vi "OP_Print_TPS20161119.vi"() -> ()   [LabVIEW 2013]
uses:
  <userlib>/caLab/Private/Get_PV-1D.vi
  <userlib>/caLab/Private/Get_PV.vi
panel:
  in  "Radio Buttons 2":enum32{"absolute", "different with"}(radio)=enum."different with"
  out "BPMY Graph":cluster{i32[], "1rst Value (number)":dbl[]}(graph)
  out "BPMX Graph":cluster{i32[], "1rst Value (number)":dbl[]}(graph)
  out "date (last Gun ON)":string="2016/08/29"
  out "time string (last Gun ON)":string="23:28:50"
  out "time string (last kicker ON)":string="23:28:50"
  out "date (last kicker ON)":string="2016/08/29"
  out "date":string="2016/08/29"
  out "time string":string="23:28:50"
  out "FOFB V":string="MBM"
  out "FOFB H":string="MBM"
  out "Value Array (number) 7":dbl[](array[numeric])=[7.29, 8.074, 40.001, 7.0, 11.0, 8.18, 40.0, 64.99985000000001, 0.0001, 65.00399999999999, 0.00055, 44.9999, 0.00025, -1.0899999999999999, 130.00060000000002]
  out "45XBPMY 1":dbl format="%#.2f"
  out "41XBPMY 1":dbl format="%#.2f"
  out "25XBPMY 1":dbl format="%#.2f"
  out "23XBPMY 1":dbl format="%#.2f"
  out "21XBPMY 1":dbl format="%#.2f"
  out "09XBPMY 1":dbl format="%#.2f"
  out "05XBPMY 1":dbl format="%#.2f"
  out "45XBPMX 1":dbl format="%#.2f"
  out "41XBPMX 1":dbl format="%#.2f"
  out "Value Array (number) 6":dbl[](array[numeric])=[7.29, 8.074, 40.001, 7.0, 11.0, 8.18, 40.0, 64.99985000000001, 0.0001, 65.00399999999999, 0.00055, 44.9999, 0.00025, -1.0899999999999999, 130.00060000000002]
  out "1rst Value (string) 2":string[](array[string])=["MBM", "33", "23.5", "350", "35.8", "22485", "22485", "62", "30", "0", "0", "160", "100"]
  out "Value Array (number) 5":dbl[](array[numeric])=[499654641.19275105, 1.0, 0.0, 1335.005102558433, 1400.0, -56.1, 1.0, 0.0, 1362.1066276040413, 1400.0, 160.0]
  out "1rst Value (string)":string[](array[string])=["Linac2016_1005_0935.data", "LTB_JT_2016_1005_1200.data", "Booster_JT_2016_1005_1200.data", "BTS_2016_1116_1020.data", "SR_DMB_2016_1102_1124LOCO.data"]
  out "Value Array (number) 4":dbl[](array[numeric])=[499654659.7918481, 1.0, 0.0, 1334.3992420266973, 1400.0, -56.70000000000001, 1.0, 0.0, 1364.2963125179533, 1400.0, 160.0]
  out "Value Array (number) 3":dbl[](array[numeric])=[0.0, 33.0, 23.5, 350.0, 35.800000000000026, 22485.0, 22485.0, 62.0, 30.0, 0.0, 0.0, 160.0, 100.0]
  out "Value Array (number) 2":dbl[](array[numeric])=[105.2, 16.40000000000001, 18.266, 18.26600000000001, 318.8444, 444.5, 419.3416, 417.0, 8.4, 8.325, 8.315, 8.27]
  out "Value Array (number)":dbl[](array[numeric])=[1.0, 302.073574, 665.9266107283645, 46.49677486881546, 27.851792365219392, 0.14677103718199608, 0.22504892367906065, 103.0465316772461, 145.84446716308594, 100.0, 630.0, 10.0]
  out "25XBPMX 1":dbl format="%#.2f"
  out "23XBPMX 1":dbl format="%#.2f"
  out "21XBPMX 1":dbl format="%#.2f"
  out "09XBPMX 1":dbl format="%#.2f"
  out "05XBPMX 1":dbl format="%#.2f"
  out "Taper":dbl=-1.0899999999999999 format="%#.4f"
  out "phase shifter":dbl=130.00060000000002 format="%#.3f"
  out "10ps delay":dbl=100.0 format="%#.1f"
  out "2ns step":dbl format="%#.1f"
  out "Width count":dbl=30.0 format="%#.1f"
  out "Gun volt.(S)":dbl=23.5 format="%#.1f"
  out "EPU46-45pM":bool
  out "EPU48B-41pM":bool
  out "EPU48A-41pM":bool
  out "IU22-05 FE Enable":bool=TRUE
  out "IU22A-09 FE Enable":bool=TRUE
  out "IUT22-21 FE Enable":bool=TRUE
  out "IU22-23 FE Enable":bool
  out "IU22A-25 FE Enable":bool=TRUE
  out "EPU48A-41 FE Enable":bool
  out "EPU46-45 FE Enable":bool=TRUE
  out "EPU46-45M Hutch Enable":bool=TRUE
  out "EPU48A-41M Hutch Enable":bool
  out "IU22A-25M Hutch Enable":bool=TRUE
  out "IU22-23M Hutch Enable":bool
  out "IUT22-21M Hutch Enable":bool=TRUE
  out "IU22A-09M Hutch Enable":bool=TRUE
  out "IU22-05 Hutch Enable":bool=TRUE
  out "Orbit ILK(P)":bool
  out "Orbit ILK(A)":bool
  out "Bucket Step":dbl=10.0 format="%#.2f"
  out "Bucket Last":dbl=630.0 format="%#.2f"
  out "Bucket Start":dbl=100.0 format="%#.2f"
  out "Orbit INT. Ang Active":bool
  out "Orbit INT.Ang. On":bool
  out "Orbit INT. Pos Active":bool
  out "Orbit INT.Pos. On":bool
  out "BR ext. kicker1":dbl=18.266 format="%#.2f"
  out "BR ext. kicker2":dbl=18.26600000000001 format="%#.2f"
  out "BR ext. sep.1":dbl=318.8444 format="%#.2f"
  out "BR ext. sep.2":dbl=444.5 format="%#.2f"
  out "BR inj. sep.":dbl=105.2 format="%#.3f"
  out "BR inj. kicker":dbl=16.40000000000001 format="%#.3f"
  out "SR kicker4":dbl=8.27 format="%#.2f"
  out "SR kicker3":dbl=8.315 format="%#.2f"
  out "SR kicker2":dbl=8.325 format="%#.2f"
  out "SR kicker1":dbl=8.4 format="%#.2f"
  out "SR inj. sep.2":dbl=417.0 format="%#.2f"
  out "SR inj. sep.1":dbl=419.3416 format="%#.2f"
  out "BBF H":bool
  out "BBF V":bool
  out "RF3 gap volt.(S)":dbl=1400.0 format="%#.0f"
  out "RF3 phase.(S)":dbl=160.0 format="%#.0f"
  out "RF3 OP mode":bool=TRUE
  out "RF3 remote":bool=TRUE
  out "RF2 gap volt.(S)":dbl=1400.0 format="%#.0f"
  out "RF Freq.(s)":dbl=499654659.7918481 format="%#.1f"
  out "RF2 phase.(S)":dbl=-56.70000000000001 format="%#.0f"
  out "RF2 OP mode":bool=TRUE
  out "RF2 remote":bool=TRUE
  out "BTS":string="SR_DMB_2016_1102_1124LOCO.data"
  out "LTB":string="LTB_JT_2016_1005_1200.data"
  out "Linac":string="Linac2016_1005_0935.data"
  out "BR":string="BTS_2016_1116_1020.data"
  out "SR":string="Booster_JT_2016_1005_1200.data"
  out "Mod.3 HV(S)":dbl=35.800000000000026 format="%#.1f"
  out "SBM volt.(S)":dbl=350.0 format="%#.1f"
  out "MBM volt.(S)":dbl=23.5 format="%#.1f"
  out "Gun mode":string="MBM"
  out "Grid volt.(S)":dbl=33.0 format="%#.1f"
  out "EPU46-45phase(R)":dbl=0.00025 format="%#.4f"
  out "EPU48B-41phase(R)":dbl=0.00055 format="%#.4f"
  out "EPU48A-41phase(R)":dbl=0.0001 format="%#.4f"
  out "EPU46-45gM":bool
  out "EPU46-45gap(R)":dbl=44.9999 format="%#.4f"
  out "EPU48B-41gM":bool
  out "EPU48B-41gap(R)":dbl=65.00399999999999 format="%#.4f"
  out "EPU48A-41gM":bool
  out "EPU48A-41gap(R)":dbl=64.99985000000001 format="%#.4f"
  out "IU22B-25M":bool
  out "IU22B-25gap(R)":dbl=40.0 format="%#.4f"
  out "IU22A-25M":bool
  out "IU22A-25gap(R)":dbl=8.18 format="%#.4f"
  out "IU22-23M":bool
  out "IUT22-21M":bool
  out "IUT22-21gap(R)":dbl=7.0 format="%#.4f"
  out "IU22B-09M":bool
  out "IU22B-09gap(R)":dbl=40.001 format="%#.4f"
  out "IU22A-09M":bool
  out "IU22A-09gap(R)":dbl=8.074 format="%#.4f"
  out "IU22-05M":bool
  out "IU22-05gap(R)":dbl=7.29 format="%#.4f"
  out "IU22-23gap(R)":dbl=11.0 format="%#.4f"
  out "NuY(form BBF)":dbl=0.25219386232318686 format="%#.2f"
  out "NuX(form BBF)":dbl=0.1781877868128751 format="%#.2f"
  out "Mode":string="Top-Up"
  out "Tune Y(form BPM)":dbl=0.2162426614481409 format="%#.2f"
  out "Tune X(form BPM)":dbl=0.14677103718199608 format="%#.2f"
  out "Beamsize Y(um)":dbl=33.47785442299371 format="%#.2f"
  out "Beamsize X(um)":dbl=55.88912339231618 format="%#.2f"
  out "Beam Lifetime(min)":dbl=665.9266107283645 format="%#.3f"
  out "Beam Current(mA":dbl=302.073574 format="%#.3f"
  in  "Copy Button":bool
  in  "Print Button":bool
  in  "Help Button":bool
  in  "Refresh Button":bool
  in  "Open Button":bool
  out "Gun WCM":dbl[](graph)
  out "BR Fill Pattern":dbl[](graph)
  out "SR Fill Pattern":dbl[](graph)
  # "Valve  Status"
  # "TPS OP Handover Information"
  # "SM Status"
  # "TPS Operational Handover Information v1.0"
  # "Time："
  # "Others"
  # "SR Status"
  # "Feedback"
  # "Pulse Mag. Status"
  # "LINAC Status"
  # "RF Status"
  # "Hz"
  # "Changeliang@BD.NSRRC"
  # "SR Fill Pattern"
  # "Lattice Files in using"
  # "歷史電流圖\ntrip次數?\n輻射劑量?\n平均氣壓\n目前最高累計劑量\n最近一次觸發時BR電流及WCM數值"
  # "ID &Beamline Status"
  # "Gap"
  # "Motor"
  # "Phase"
  # "FE/Hutch"
  # "phase\nshifter"
  # "Taper"
  # "XBPM1X\num"
  # "XBPM1Y\num"
  # "05"
  # "09"
  # "21"
  # "23"
  # "25"
  # "41"
  # "45"
  # "SR Orbit"
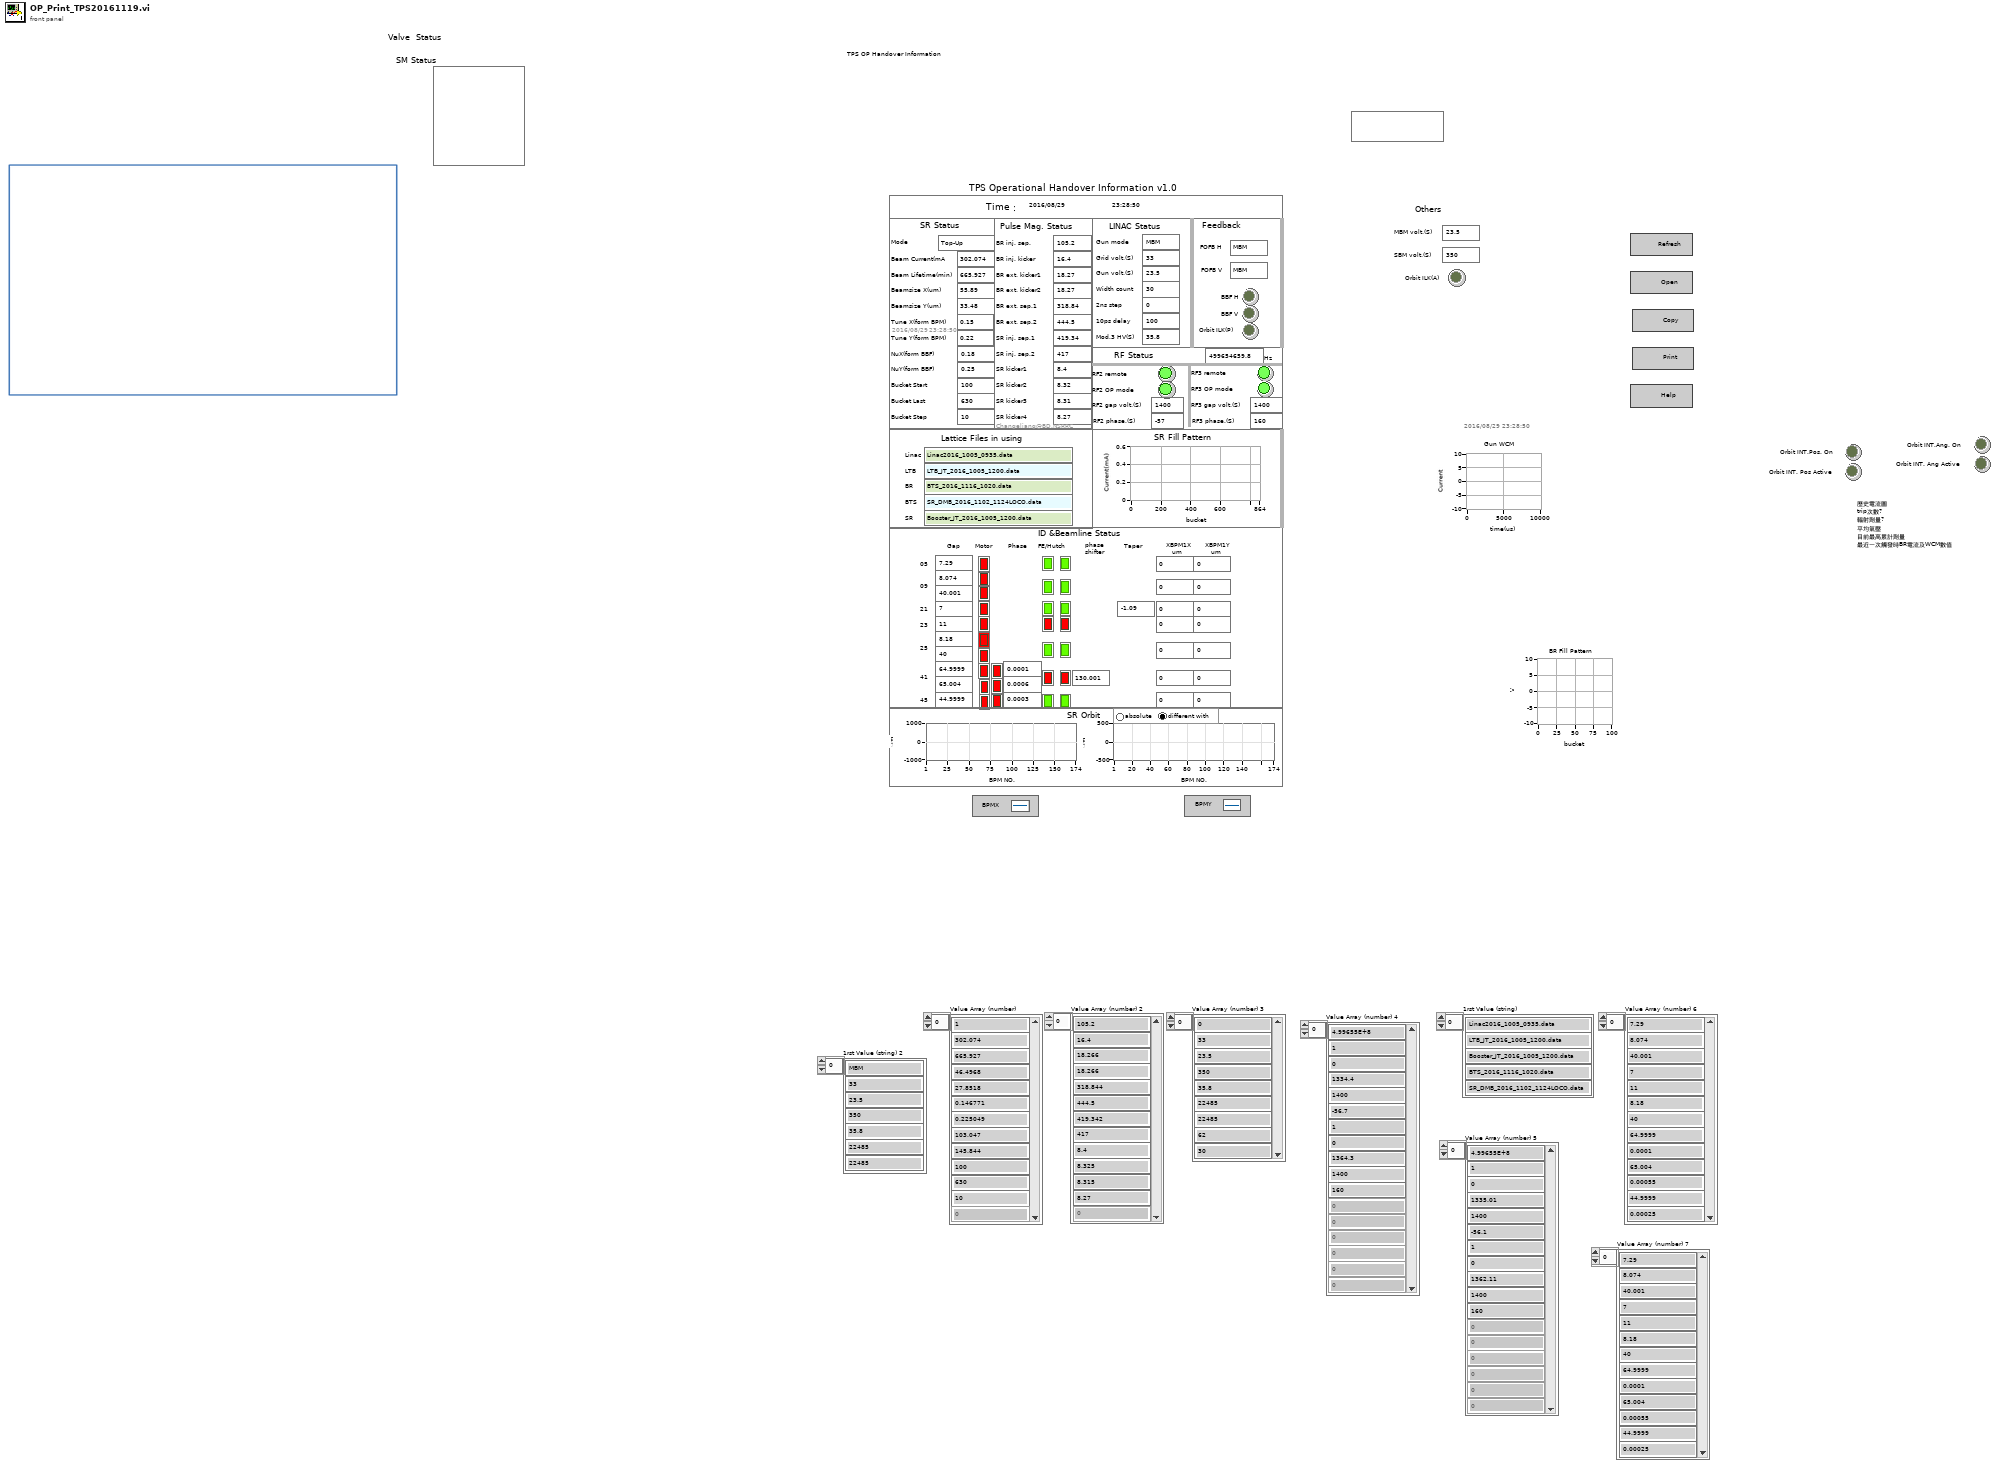
[diagram p1: front panel]
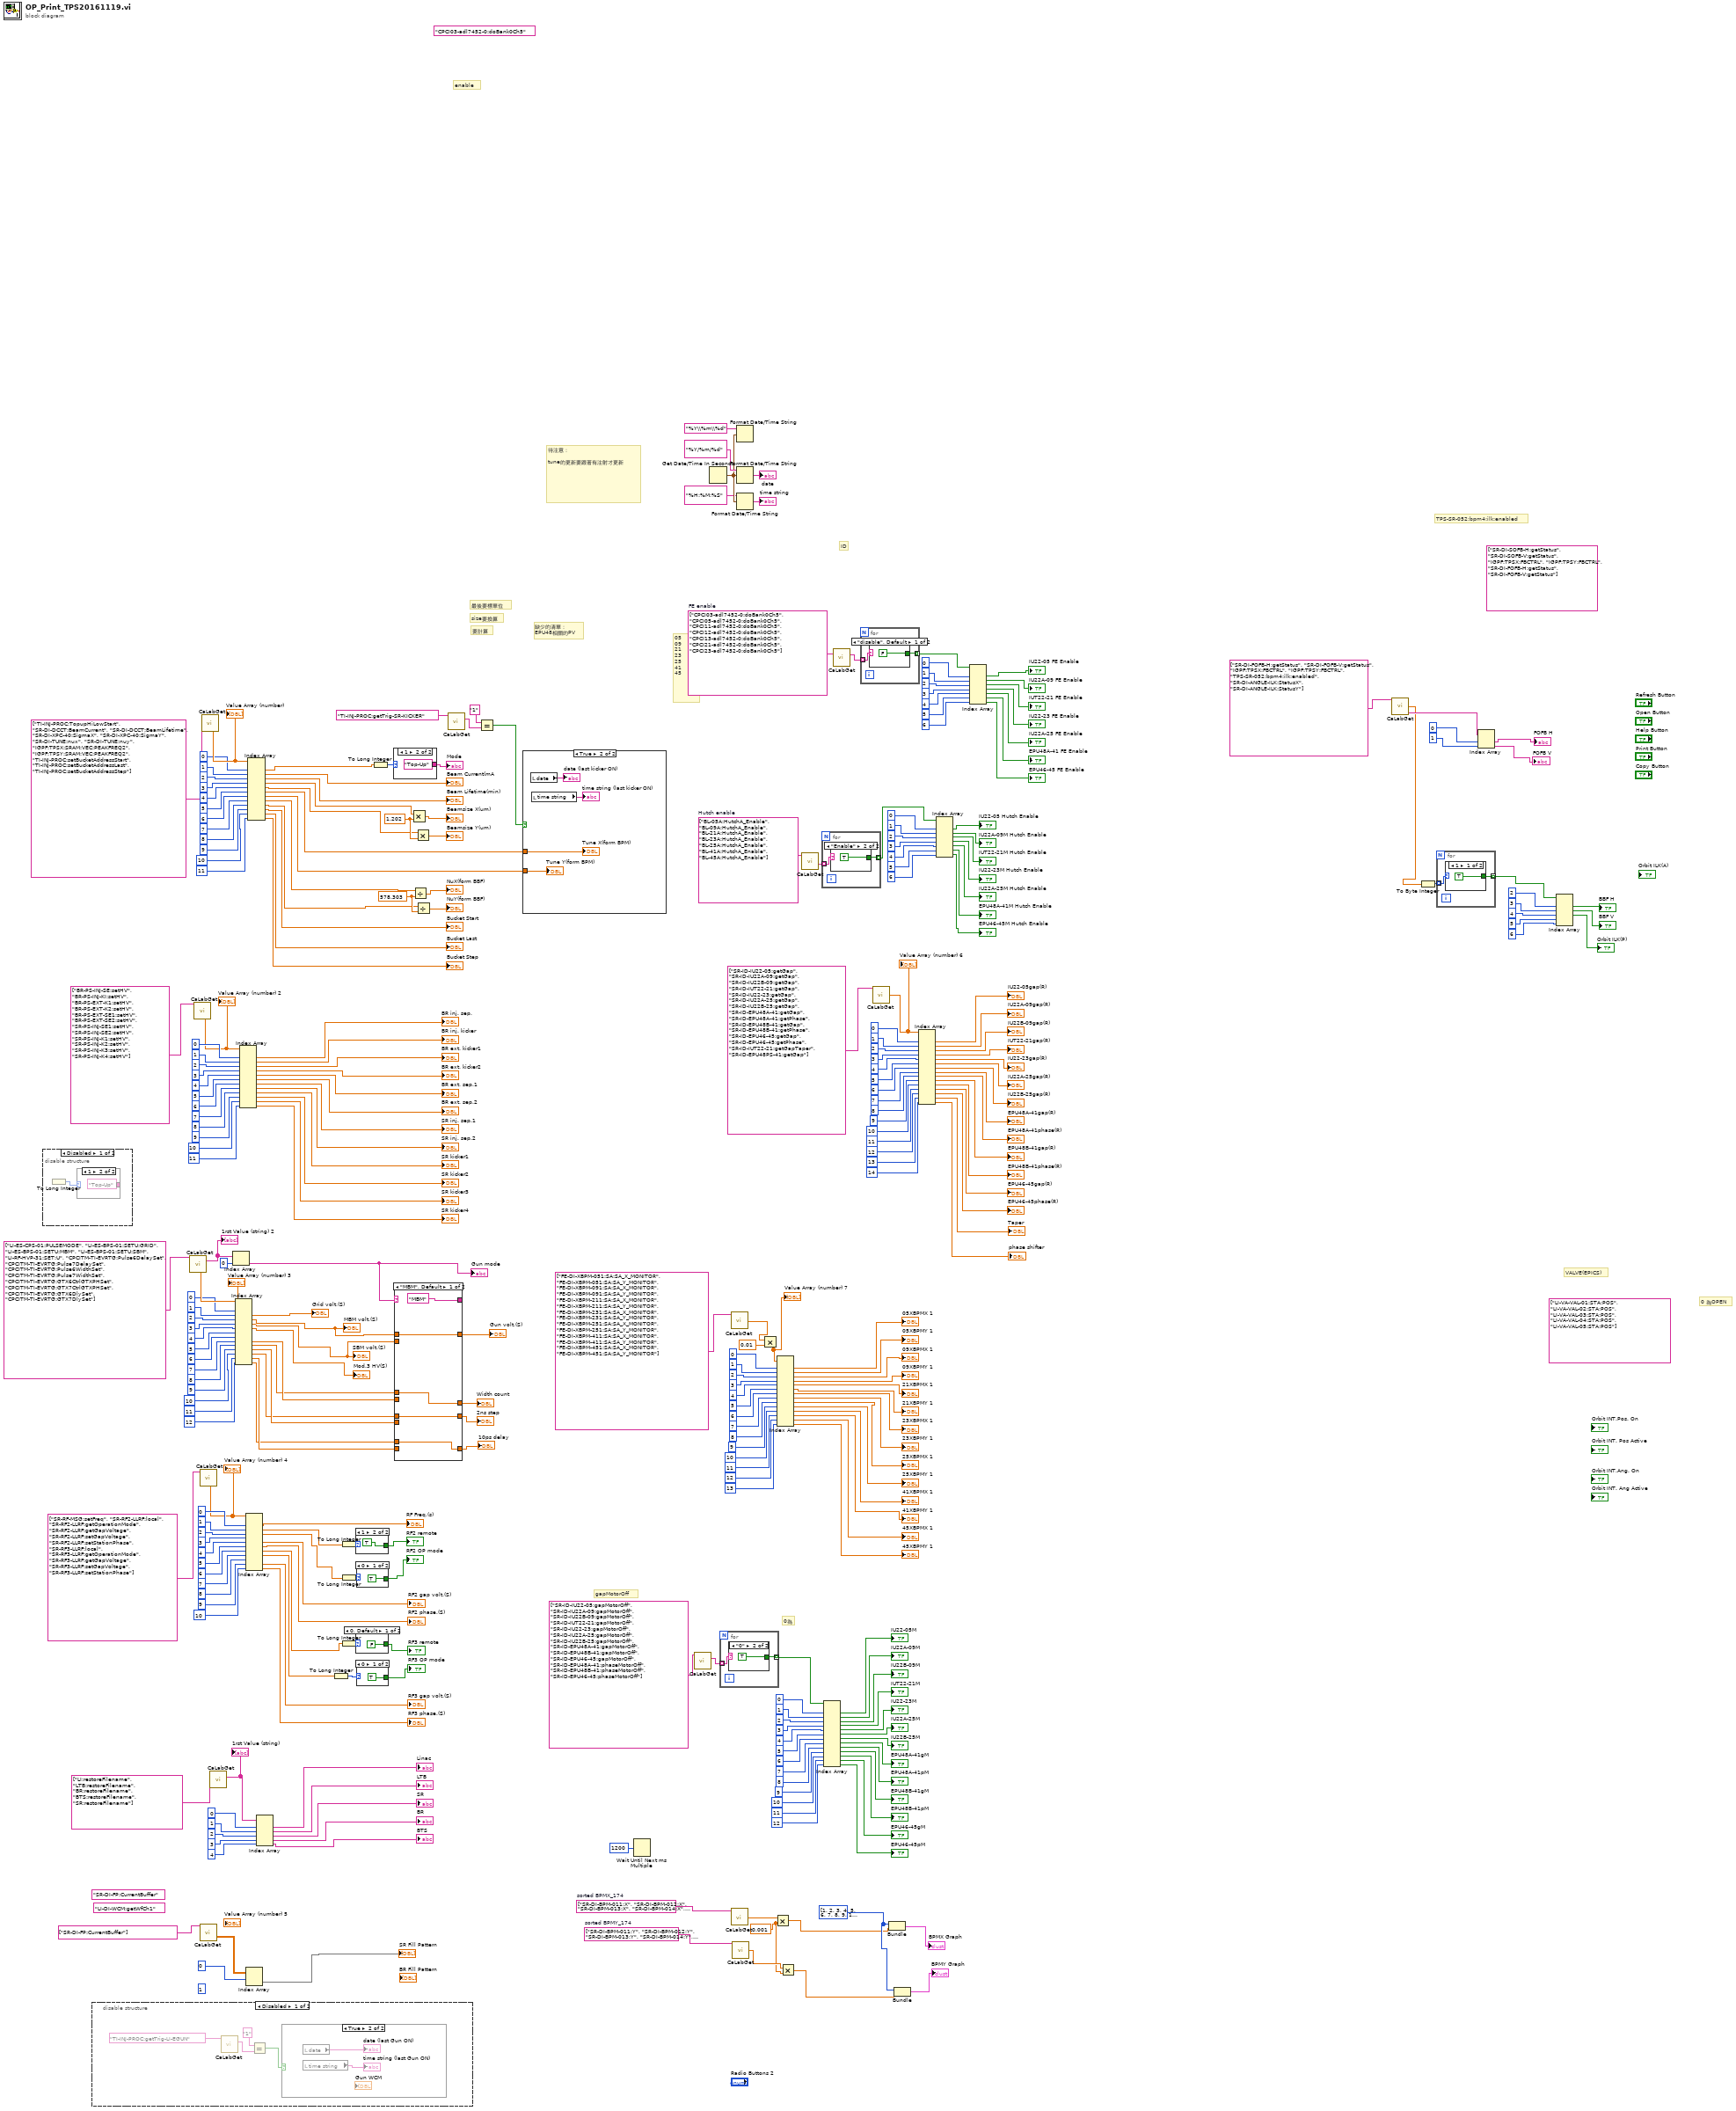
[diagram p0: block diagram]
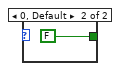
[diagram p4: hidden frame]
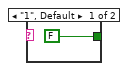
[diagram p5: hidden frame]
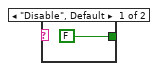
[diagram p6: hidden frame]
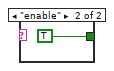
[diagram p7: hidden frame]
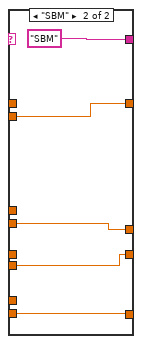
[diagram p8: hidden frame]
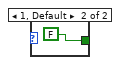
[diagram p10: hidden frame]
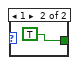
[diagram p11: hidden frame]
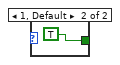
[diagram p12: hidden frame]
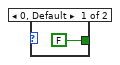
[diagram p13: hidden frame]
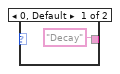
[diagram p14: hidden frame]
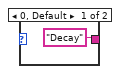
[diagram p16: hidden frame]
diagram:
  (unwired) "LI-DI-WCM:getWfCh1"
  (unwired) "SR-DI-FP:CurrentBuffer"
  w12 = i32[] [1, 2, 3, 4, 5, 6, 7, 8, 9, 10, 11, 12, 13, 14, 15, 16, 17, 18, 19, 20, 21, 22, 23, 24, 25, 26, 27, 28, 29, 30, 31, 32, 33, 34, 35, 36, 37, 38, 39, 40, 41, 42, 43, 44, 45, 46, 47, 48, 49, 50, 51, 52, 53, 54, 55, 56, 57, 58, 59, 60, 61, 62, 63, 64, 65, 66, 67, 68, 69, 70, 71, 72, 73, 74, 75, 76, 77, 78, 79, 80, 81, 82, 83, 84, 85, 86, 87, 88, 89, 90, 91, 92, 93, 94, 95, 96, 97, 98, 99, 100, 101, 102, 103, 104, 105, 106, 107, 108, 109, 110, 111, 112, 113, 114, 115, 116, 117, 118, 119, 120, 121, 122, 123, 124, 125, 126, 127, 128, 129, 130, 131, 132, 133, 134, 135, 136, 137, 138, 139, 140, 141, 142, 143, 144, 145, 146, 147, 148, 149, 150, 151, 152, 153, 154, 155, 156, 157, 158, 159, 160, 161, 162, 163, 164, 165, 166, 167, 168, 169, 170, 171, 172, 173, 174] ("Array 4")
  w9 = 0.001
  w6 = string[] ["SR-DI-BPM-011:Y", "SR-DI-BPM-012:Y", "SR-DI-BPM-013:Y", "SR-DI-BPM-014:Y", "SR-DI-BPM-015:Y", "SR-DI-BPM-016:Y", "SR-DI-BPM-017:Y", "SR-DI-BPM-021:Y", "SR-DI-BPM-022:Y", "SR-DI-BPM-023:Y", "SR-DI-BPM-024:Y", "SR-DI-BPM-025:Y", "SR-DI-BPM-026:Y", "SR-DI-BPM-027:Y", "SR-DI-BPM-031:Y", "SR-DI-BPM-032:Y", "SR-DI-BPM-033:Y", "SR-DI-BPM-034:Y", "SR-DI-BPM-035:Y", "SR-DI-BPM-036:Y", "SR-DI-BPM-037:Y", "SR-DI-BPM-041:Y", "SR-DI-BPM-042:Y", "SR-DI-BPM-043:Y", "SR-DI-BPM-044:Y", "SR-DI-BPM-045:Y", "SR-DI-BPM-046:Y", "SR-DI-BPM-047:Y", "SR-DI-BPM-048:Y", "SR-DI-BPM-050:Y", "SR-DI-BPM-051:Y", "SR-DI-BPM-052:Y", "SR-DI-BPM-053:Y", "SR-DI-BPM-054:Y", "SR-DI-BPM-055:Y", "SR-DI-BPM-056:Y", "SR-DI-BPM-057:Y", "SR-DI-BPM-061:Y", "SR-DI-BPM-062:Y", "SR-DI-BPM-063:Y", "SR-DI-BPM-064:Y", "SR-DI-BPM-065:Y", "SR-DI-BPM-066:Y", "SR-DI-BPM-067:Y", "SR-DI-BPM-071:Y", "SR-DI-BPM-072:Y", "SR-DI-BPM-073:Y", "SR-DI-BPM-074:Y", "SR-DI-BPM-075:Y", "SR-DI-BPM-076:Y", "SR-DI-BPM-077:Y", "SR-DI-BPM-081:Y", "SR-DI-BPM-082:Y", "SR-DI-BPM-083:Y", "SR-DI-BPM-084:Y", "SR-DI-BPM-085:Y", "SR-DI-BPM-086:Y", "SR-DI-BPM-087:Y", "SR-DI-BPM-091:Y", "SR-DI-BPM-092:Y", "SR-DI-BPM-093:Y", "SR-DI-BPM-094:Y", "SR-DI-BPM-095:Y", "SR-DI-BPM-096:Y", "SR-DI-BPM-097:Y", "SR-DI-BPM-101:Y", "SR-DI-BPM-102:Y", "SR-DI-BPM-103:Y", "SR-DI-BPM-104:Y", "SR-DI-BPM-105:Y", "SR-DI-BPM-106:Y", "SR-DI-BPM-107:Y", "SR-DI-BPM-111:Y", "SR-DI-BPM-112:Y", "SR-DI-BPM-113:Y", "SR-DI-BPM-114:Y", "SR-DI-BPM-115:Y", "SR-DI-BPM-116:Y", "SR-DI-BPM-117:Y", "SR-DI-BPM-121:Y", "SR-DI-BPM-122:Y", "SR-DI-BPM-123:Y", "SR-DI-BPM-124:Y", "SR-DI-BPM-125:Y", "SR-DI-BPM-126:Y", "SR-DI-BPM-127:Y", "SR-DI-BPM-128:Y", "SR-DI-BPM-130:Y", "SR-DI-BPM-131:Y", "SR-DI-BPM-132:Y", "SR-DI-BPM-133:Y", "SR-DI-BPM-134:Y", "SR-DI-BPM-135:Y", "SR-DI-BPM-136:Y", "SR-DI-BPM-137:Y", "SR-DI-BPM-141:Y", "SR-DI-BPM-142:Y", "SR-DI-BPM-143:Y", "SR-DI-BPM-144:Y", "SR-DI-BPM-145:Y", "SR-DI-BPM-146:Y", "SR-DI-BPM-147:Y", "SR-DI-BPM-151:Y", "SR-DI-BPM-152:Y", "SR-DI-BPM-153:Y", "SR-DI-BPM-154:Y", "SR-DI-BPM-155:Y", "SR-DI-BPM-156:Y", "SR-DI-BPM-157:Y", "SR-DI-BPM-161:Y", "SR-DI-BPM-162:Y", "SR-DI-BPM-163:Y", "SR-DI-BPM-164:Y", "SR-DI-BPM-165:Y", "SR-DI-BPM-166:Y", "SR-DI-BPM-167:Y", "SR-DI-BPM-171:Y", "SR-DI-BPM-172:Y", "SR-DI-BPM-173:Y", "SR-DI-BPM-174:Y", "SR-DI-BPM-175:Y", "SR-DI-BPM-176:Y", "SR-DI-BPM-177:Y", "SR-DI-BPM-181:Y", "SR-DI-BPM-182:Y", "SR-DI-BPM-183:Y", "SR-DI-BPM-184:Y", "SR-DI-BPM-185:Y", "SR-DI-BPM-186:Y", "SR-DI-BPM-187:Y", "SR-DI-BPM-191:Y", "SR-DI-BPM-192:Y", "SR-DI-BPM-193:Y", "SR-DI-BPM-194:Y", "SR-DI-BPM-195:Y", "SR-DI-BPM-196:Y", "SR-DI-BPM-197:Y", "SR-DI-BPM-201:Y", "SR-DI-BPM-202:Y", "SR-DI-BPM-203:Y", "SR-DI-BPM-204:Y", "SR-DI-BPM-205:Y", "SR-DI-BPM-206:Y", "SR-DI-BPM-207:Y", "SR-DI-BPM-208:Y", "SR-DI-BPM-210:Y", "SR-DI-BPM-211:Y", "SR-DI-BPM-212:Y", "SR-DI-BPM-213:Y", "SR-DI-BPM-214:Y", "SR-DI-BPM-215:Y", "SR-DI-BPM-216:Y", "SR-DI-BPM-217:Y", "SR-DI-BPM-221:Y", "SR-DI-BPM-222:Y", "SR-DI-BPM-223:Y", "SR-DI-BPM-224:Y", "SR-DI-BPM-225:Y", "SR-DI-BPM-226:Y", "SR-DI-BPM-227:Y", "SR-DI-BPM-231:Y", "SR-DI-BPM-232:Y", "SR-DI-BPM-233:Y", "SR-DI-BPM-234:Y", "SR-DI-BPM-235:Y", "SR-DI-BPM-236:Y", "SR-DI-BPM-237:Y", "SR-DI-BPM-241:Y", "SR-DI-BPM-242:Y", "SR-DI-BPM-243:Y", "SR-DI-BPM-244:Y", "SR-DI-BPM-245:Y", "SR-DI-BPM-246:Y", "SR-DI-BPM-247:Y"]  # sorted BPMY_174
  w5 = string[] ["SR-DI-BPM-011:X", "SR-DI-BPM-012:X", "SR-DI-BPM-013:X", "SR-DI-BPM-014:X", "SR-DI-BPM-015:X", "SR-DI-BPM-016:X", "SR-DI-BPM-017:X", "SR-DI-BPM-021:X", "SR-DI-BPM-022:X", "SR-DI-BPM-023:X", "SR-DI-BPM-024:X", "SR-DI-BPM-025:X", "SR-DI-BPM-026:X", "SR-DI-BPM-027:X", "SR-DI-BPM-031:X", "SR-DI-BPM-032:X", "SR-DI-BPM-033:X", "SR-DI-BPM-034:X", "SR-DI-BPM-035:X", "SR-DI-BPM-036:X", "SR-DI-BPM-037:X", "SR-DI-BPM-041:X", "SR-DI-BPM-042:X", "SR-DI-BPM-043:X", "SR-DI-BPM-044:X", "SR-DI-BPM-045:X", "SR-DI-BPM-046:X", "SR-DI-BPM-047:X", "SR-DI-BPM-048:X", "SR-DI-BPM-050:X", "SR-DI-BPM-051:X", "SR-DI-BPM-052:X", "SR-DI-BPM-053:X", "SR-DI-BPM-054:X", "SR-DI-BPM-055:X", "SR-DI-BPM-056:X", "SR-DI-BPM-057:X", "SR-DI-BPM-061:X", "SR-DI-BPM-062:X", "SR-DI-BPM-063:X", "SR-DI-BPM-064:X", "SR-DI-BPM-065:X", "SR-DI-BPM-066:X", "SR-DI-BPM-067:X", "SR-DI-BPM-071:X", "SR-DI-BPM-072:X", "SR-DI-BPM-073:X", "SR-DI-BPM-074:X", "SR-DI-BPM-075:X", "SR-DI-BPM-076:X", "SR-DI-BPM-077:X", "SR-DI-BPM-081:X", "SR-DI-BPM-082:X", "SR-DI-BPM-083:X", "SR-DI-BPM-084:X", "SR-DI-BPM-085:X", "SR-DI-BPM-086:X", "SR-DI-BPM-087:X", "SR-DI-BPM-091:X", "SR-DI-BPM-092:X", "SR-DI-BPM-093:X", "SR-DI-BPM-094:X", "SR-DI-BPM-095:X", "SR-DI-BPM-096:X", "SR-DI-BPM-097:X", "SR-DI-BPM-101:X", "SR-DI-BPM-102:X", "SR-DI-BPM-103:X", "SR-DI-BPM-104:X", "SR-DI-BPM-105:X", "SR-DI-BPM-106:X", "SR-DI-BPM-107:X", "SR-DI-BPM-111:X", "SR-DI-BPM-112:X", "SR-DI-BPM-113:X", "SR-DI-BPM-114:X", "SR-DI-BPM-115:X", "SR-DI-BPM-116:X", "SR-DI-BPM-117:X", "SR-DI-BPM-121:X", "SR-DI-BPM-122:X", "SR-DI-BPM-123:X", "SR-DI-BPM-124:X", "SR-DI-BPM-125:X", "SR-DI-BPM-126:X", "SR-DI-BPM-127:X", "SR-DI-BPM-128:X", "SR-DI-BPM-130:X", "SR-DI-BPM-131:X", "SR-DI-BPM-132:X", "SR-DI-BPM-133:X", "SR-DI-BPM-134:X", "SR-DI-BPM-135:X", "SR-DI-BPM-136:X", "SR-DI-BPM-137:X", "SR-DI-BPM-141:X", "SR-DI-BPM-142:X", "SR-DI-BPM-143:X", "SR-DI-BPM-144:X", "SR-DI-BPM-145:X", "SR-DI-BPM-146:X", "SR-DI-BPM-147:X", "SR-DI-BPM-151:X", "SR-DI-BPM-152:X", "SR-DI-BPM-153:X", "SR-DI-BPM-154:X", "SR-DI-BPM-155:X", "SR-DI-BPM-156:X", "SR-DI-BPM-157:X", "SR-DI-BPM-161:X", "SR-DI-BPM-162:X", "SR-DI-BPM-163:X", "SR-DI-BPM-164:X", "SR-DI-BPM-165:X", "SR-DI-BPM-166:X", "SR-DI-BPM-167:X", "SR-DI-BPM-171:X", "SR-DI-BPM-172:X", "SR-DI-BPM-173:X", "SR-DI-BPM-174:X", "SR-DI-BPM-175:X", "SR-DI-BPM-176:X", "SR-DI-BPM-177:X", "SR-DI-BPM-181:X", "SR-DI-BPM-182:X", "SR-DI-BPM-183:X", "SR-DI-BPM-184:X", "SR-DI-BPM-185:X", "SR-DI-BPM-186:X", "SR-DI-BPM-187:X", "SR-DI-BPM-191:X", "SR-DI-BPM-192:X", "SR-DI-BPM-193:X", "SR-DI-BPM-194:X", "SR-DI-BPM-195:X", "SR-DI-BPM-196:X", "SR-DI-BPM-197:X", "SR-DI-BPM-201:X", "SR-DI-BPM-202:X", "SR-DI-BPM-203:X", "SR-DI-BPM-204:X", "SR-DI-BPM-205:X", "SR-DI-BPM-206:X", "SR-DI-BPM-207:X", "SR-DI-BPM-208:X", "SR-DI-BPM-210:X", "SR-DI-BPM-211:X", "SR-DI-BPM-212:X", "SR-DI-BPM-213:X", "SR-DI-BPM-214:X", "SR-DI-BPM-215:X", "SR-DI-BPM-216:X", "SR-DI-BPM-217:X", "SR-DI-BPM-221:X", "SR-DI-BPM-222:X", "SR-DI-BPM-223:X", "SR-DI-BPM-224:X", "SR-DI-BPM-225:X", "SR-DI-BPM-226:X", "SR-DI-BPM-227:X", "SR-DI-BPM-231:X", "SR-DI-BPM-232:X", "SR-DI-BPM-233:X", "SR-DI-BPM-234:X", "SR-DI-BPM-235:X", "SR-DI-BPM-236:X", "SR-DI-BPM-237:X", "SR-DI-BPM-241:X", "SR-DI-BPM-242:X", "SR-DI-BPM-243:X", "SR-DI-BPM-244:X", "SR-DI-BPM-245:X", "SR-DI-BPM-246:X", "SR-DI-BPM-247:X"]  # sorted BPMX_174
  w136 = string[] ["BL-05A:HutchA_Enable", "BL-09A:HutchA_Enable", "BL-21A:HutchA_Enable", "BL-23A:HutchA_Enable", "BL-25A:HutchA_Enable", "BL-41A:HutchA_Enable", "BL-45A:HutchA_Enable"]  # Hutch enable
  (unwired) "CPCI03-adl7452-0:doBank0Ch5"
  w162 = string[] ["CPCI03-adl7452-0:doBank0Ch5", "CPCI05-adl7452-0:doBank0Ch5", "CPCI11-adl7452-0:doBank0Ch5", "CPCI12-adl7452-0:doBank0Ch5", "CPCI13-adl7452-0:doBank0Ch5", "CPCI21-adl7452-0:doBank0Ch5", "CPCI23-adl7452-0:doBank0Ch5"]  # FE enable
  (unwired) 1 ("index")
  w275 = 578.303 ("y")
  w282 = 1.202 ("y")
  (unwired) string[] ["LI-VA-VAL-01:STA:POS", "LI-VA-VAL-02:STA:POS", "LI-VA-VAL-03:STA:POS", "LI-VA-VAL-04:STA:POS", "LI-VA-VAL-05:STA:POS"]
  (unwired) string[] ["SR-DI-SOFB-H:getStatus", "SR-DI-SOFB-V:getStatus", "IGPF:TPSX:FBCTRL", "IGPF:TPSY:FBCTRL", "SR-DI-FOFB-H:getStatus", "SR-DI-FOFB-V:getStatus"]
  # "TPS-SR-052:bpm4:ilk:enabled"
  # "0為"
  # "ID"
  # "05\n09\n21\n23\n25\n41\n45"
  # "enable"
  # "待注意：\n\ntune的更新要跟著有注射才更新"
  # "0 為OPEN"
  # "VALVE(EPICS)"
  # "要計算"
  # "gapMotorOff"
  # "最後要標單位"
  # "size要換算"
  # "缺少的清單：\nEPU48相關的PV"
  n1 = disable-structure shown="Disabled" {
    frame Disabled {
      n2 = To Long Integer() -> (32bit integer=w304:i32)  [unwired: 1 in]
      n3 = case shown="1" w304 {
        tunnel: ["Decay" "Top-Up"] -> _
        frame 0, Default {
        }
        frame 1 {
        }
      }
    }
    frame Enabled {
    }
  }
  n4 = disable-structure shown="Disabled" {
    frame Disabled {
      n5 = call-poly <userlib>:"CaLabGet.vi"("PV Name"="TI-INJ-PROC:getTrig-LI-EGUN") -> ("1rst Value (string)"=w309:string)  [unwired: 8 in, 6 out]
      n6 = Equal?(x="1" ("1rst Value (string)"), y=w309) -> (x = y?=w307:bool)
      n7 = case shown="True" w307 {
        frame False {
        }
        frame True {
          n8 = local read "date"() -> (→"date (last Gun ON)":string)
          n9 = local read "time string"() -> (→"time string (last Gun ON)":string)
        }
      }
    }
    frame Enabled {
    }
  }
  n10 = call-poly <userlib>:"CaLabGet.vi"("PV Names"=string[] ["LI-ES-CPS-01:PULSEMODE", "LI-ES-BPS-01:SETU:GRID", "LI-ES-BPS-01:SETU:MBM", "LI-ES-BPS-01:SETU:SBM", "LI-RF-HVP-31:SET:U", "CPCITM-TI-EVRTG:Pulse6DelaySet", "CPCITM-TI-EVRTG:Pulse7DelaySet", "CPCITM-TI-EVRTG:Pulse6WidthSet", "CPCITM-TI-EVRTG:Pulse7WidthSet", "CPCITM-TI-EVRTG:GTX6CtrlGTXPHSet", "CPCITM-TI-EVRTG:GTX7CtrlGTXPHSet", "CPCITM-TI-EVRTG:GTX6DlySet", "CPCITM-TI-EVRTG:GTX7DlySet"]) -> ("1rst Value (string)"=w175:string[], "1rst Value (number)"=w243:dbl[])  [unwired: 8 in, 5 out]
  "Value Array (number) 3" <- w243
  "1rst Value (string) 2" <- w175
  n11 = call-poly <userlib>:"CaLabGet.vi"("PV Names"=string[] ["BR-PS-INJ-SE:setHV", "BR-PS-INJ-KI:setHV", "BR-PS-EXT-K1:setHV", "BR-PS-EXT-K2:setHV", "BR-PS-EXT-SE1:setHV", "BR-PS-EXT-SE2:setHV", "SR-PS-INJ-SE1:setHV", "SR-PS-INJ-SE2:setHV", "SR-PS-INJ-K1:setHV", "SR-PS-INJ-K2:setHV", "SR-PS-INJ-K3:setHV", "SR-PS-INJ-K4:setHV"]) -> ("1rst Value (number)"=w257:dbl[])  [unwired: 8 in, 6 out]
  "Value Array (number) 2" <- w257
  n12 = call-poly <userlib>:"CaLabGet.vi"("PV Names"=string[] ["SR-RF-MSG:setFreq", "SR-RF2-LLRF:local", "SR-RF2-LLRF:getOperationMode", "SR-RF2-LLRF:getGapVoltage", "SR-RF2-LLRF:setGapVoltage", "SR-RF2-LLRF:setStationPhase", "SR-RF3-LLRF:local", "SR-RF3-LLRF:getOperationMode", "SR-RF3-LLRF:getGapVoltage", "SR-RF3-LLRF:setGapVoltage", "SR-RF3-LLRF:setStationPhase"]) -> ("1rst Value (number)"=w218:dbl[])  [unwired: 8 in, 6 out]
  "Value Array (number) 4" <- w218
  n13 = call-poly <userlib>:"CaLabGet.vi"("PV Names"=string[] ["SR-DI-FP:CurrentBuffer"]) -> ("Value Array (number)"=w186:dbl[][])  [unwired: 8 in, 6 out]
  n14 = call-poly <userlib>:"CaLabGet.vi"("PV Names"=string[] ["TI-INJ-PROC:TopupHiLowStart", "SR-DI-DCCT:BeamCurrent", "SR-DI-DCCT:BeamLifetime", "SR-DI-XPC-40:SigmaX", "SR-DI-XPC-40:SigmaY", "SR-DI-TUNE:nux", "SR-DI-TUNE:nuy", "IGPF:TPSX:SRAM:VEC:PEAKFREQ2", "IGPF:TPSY:SRAM:VEC:PEAKFREQ2", "TI-INJ-PROC:setBucketAddressStart", "TI-INJ-PROC:setBucketAddressLast", "TI-INJ-PROC:setBucketAddressStep"]) -> ("1rst Value (number)"=w300:dbl[])  [unwired: 8 in, 6 out]
  "Value Array (number)" <- w300
  n15 = call-poly <userlib>:"CaLabGet.vi"("PV Names"=string[] ["LI:restoreFilename", "LTB:restoreFilename", "BR:restoreFilename", "BTS:restoreFilename", "SR:restoreFilename"]) -> ("1rst Value (string)"=w193:string[])  [unwired: 8 in, 6 out]
  "1rst Value (string)" <- w193
  n16 = Index Array(array=w175, index=0) -> (element=w173:string)
  "Gun mode" <- w173
  n17 = Index Array(array=w243, index #1=0 ("index"), index #2=1 ("index"), index #3=2 ("index"), index #4=3 ("index"), index #5=4 ("index"), index #6=5 ("index"), index #7=6 ("index"), index #8=7 ("index"), index #9=8 ("index"), index #10=9 ("index"), index #11=10 ("index"), index #12=11 ("index"), index #13=12 ("index")) -> (element #2=→"Grid volt.(S)":dbl, element #3=w179:dbl, element #4=w178:dbl, element #5=→"Mod.3 HV(S)":dbl, element #8=w172:dbl, element #9=w171:dbl, element #10=w169:dbl, element #11=w168:dbl, element #12=w166:dbl, element #13=w165:dbl)  [unwired: 3 out]
  "MBM volt.(S)" <- w179
  "SBM volt.(S)" <- w178
  n18 = Index Array(array=w257, index #1=0 ("index"), index #2=1 ("index"), index #3=2 ("index"), index #4=3 ("index"), index #5=4 ("index"), index #6=5 ("index"), index #7=6 ("index"), index #8=7 ("index"), index #9=8 ("index"), index #10=9 ("index"), index #11=10 ("index"), index #12=11 ("index")) -> (element #1=→"BR inj. sep.":dbl, element #2=→"BR inj. kicker":dbl, element #3=→"BR ext. kicker1":dbl, element #4=→"BR ext. kicker2":dbl, element #5=→"BR ext. sep.1":dbl, element #6=→"BR ext. sep.2":dbl, element #7=→"SR inj. sep.1":dbl, element #8=→"SR inj. sep.2":dbl, element #9=→"SR kicker1":dbl, element #10=→"SR kicker2":dbl, element #11=→"SR kicker3":dbl, element #12=→"SR kicker4":dbl)
  n19 = Index Array(array=w218, index #1=0 ("index"), index #2=1 ("index"), index #3=2 ("index"), index #4=3 ("index"), index #5=4 ("index"), index #6=5 ("index"), index #7=6 ("index"), index #8=7 ("index"), index #9=8 ("index"), index #10=9 ("index"), index #11=10 ("index")) -> (element #1=→"RF Freq.(s)":dbl, element #2=w213:dbl, element #3=w210:dbl, element #5=→"RF2 gap volt.(S)":dbl, element #6=→"RF2 phase.(S)":dbl, element #7=w205:dbl, element #8=w204:dbl, element #10=→"RF3 gap volt.(S)":dbl, element #11=→"RF3 phase.(S)":dbl)  [unwired: 2 out]
  n20 = Index Array(array=w186, index (row)=0 ("index")) -> (element=→"SR Fill Pattern":dbl[])  [unwired: 1 in]
  n21 = Index Array(array=w300, index #1=0 ("index"), index #2=1 ("index"), index #3=2 ("index"), index #4=3 ("index"), index #5=4 ("index"), index #6=5 ("index"), index #7=6 ("index"), index #8=7 ("index"), index #9=8 ("index"), index #10=9 ("index"), index #11=10 ("index"), index #12=11 ("index")) -> (element #1=w298:dbl, element #2=→"Beam Current(mA":dbl, element #3=→"Beam Lifetime(min)":dbl, element #4=w283:dbl, element #5=w281:dbl, element #6=w280:dbl, element #7=w278:dbl, element #8=w277:dbl, element #9=w274:dbl, element #10=→"Bucket Start":dbl, element #11=→"Bucket Last":dbl, element #12=→"Bucket Step":dbl)
  n22 = Index Array(array=w193, index #1=0 ("index"), index #2=1 ("index"), index #3=2 ("index"), index #4=3 ("index"), index #5=4 ("index")) -> (element #1=→"Linac":string, element #2=→"LTB":string, element #3=→"SR":string, element #4=→"BR":string, element #5=→"BTS":string)
  n23 = To Long Integer(number=w204) -> (32bit integer=w207:i32)
  n24 = To Long Integer(number=w213) -> (32bit integer=w215:i32)
  n25 = To Long Integer(number=w205) -> (32bit integer=w206:i32)
  n26 = To Long Integer(number=w210) -> (32bit integer=w212:i32)
  n27 = case shown="1" w215 {
    tunnel: [FALSE TRUE] -> w214
    frame 0, Default {
    }
    frame 1 {
    }
  }
  "RF2 remote" <- w214
  n28 = case shown="0, Default" w206 {
    tunnel: [FALSE TRUE] -> w202
    frame 0, Default {
    }
    frame 1 {
    }
  }
  "RF3 remote" <- w202
  n29 = case shown="0" w212 {
    tunnel: [TRUE TRUE] -> w211
    frame 0 {
    }
    frame 1, Default {
    }
  }
  "RF2 OP mode" <- w211
  n30 = case shown="0" w207 {
    tunnel: [TRUE FALSE] -> w203
    frame 0 {
    }
    frame 1, Default {
    }
  }
  "RF3 OP mode" <- w203
  n31 = To Long Integer(number=w298) -> (32bit integer=w301:i32)
  n32 = case shown="1" w301 {
    tunnel: ["Decay" "Top-Up"] -> w302
    frame 0, Default {
    }
    frame 1 {
    }
  }
  "Mode" <- w302
  n33 = case shown="\"MBM\", Default" w173 {
    tunnel: ["MBM" "SBM"] -> _
    tunnel: w179 -> [w326 _]
    tunnel: [w326 w331] -> w177
    tunnel: w178 -> [_ w331]
    tunnel: w172 -> [_ w330]
    tunnel: w171 -> [w325 _]
    tunnel: [w325 w330] -> w170
    tunnel: w169 -> [_ w329]
    tunnel: w168 -> [w324 _]
    tunnel: [w324 w329] -> w167
    tunnel: w166 -> [_ w328]
    tunnel: w165 -> [w323 _]
    tunnel: [w323 w328] -> w164
    frame "MBM", Default {
    }
    frame "SBM" {
    }
  }
  "Gun volt.(S)" <- w177
  "Width count" <- w170
  "2ns step" <- w167
  "10ps delay" <- w164
  n34 = Multiply(x=w283, y=w282) -> (x*y=→"Beamsize X(um)":dbl)
  n35 = Divide(x=w277, y=w275) -> (x/y=→"NuX(form BBF)":dbl)
  n36 = Multiply(x=w281, y=w282) -> (x*y=→"Beamsize Y(um)":dbl)
  n37 = Divide(x=w274, y=w275) -> (x/y=→"NuY(form BBF)":dbl)
  n38 = call-poly <userlib>:"CaLabGet.vi"("PV Name"="TI-INJ-PROC:getTrig-SR-KICKER") -> ("1rst Value (string)"=w183:string)  [unwired: 8 in, 6 out]
  n39 = Equal?(x="1" ("1rst Value (string)"), y=w183) -> (x = y?=w181:bool)
  n40 = case shown="True" w181 {
    tunnel: w280 -> [_ w336]
    tunnel: w278 -> [_ w335]
    frame False {
    }
    frame True {
      n41 = local read "date"() -> (→"date (last kicker ON)":string)
      n42 = local read "time string"() -> (→"time string (last kicker ON)":string)
      "Tune X(form BPM)" <- w336
      "Tune Y(form BPM)" <- w335
    }
  }
  n43 = Wait Until Next ms Multiple(millisecond multiple=u32 1200) -> ()  [unwired: 1 out]
  n44 = call-poly <userlib>:"CaLabGet.vi"("PV Names"=string[] ["SR-ID-IU22-05:gapMotorOff", "SR-ID-IU22A-09:gapMotorOff", "SR-ID-IU22B-09:gapMotorOff", "SR-ID-IUT22-21:gapMotorOff", "SR-ID-IU22-23:gapMotorOff", "SR-ID-IU22A-25:gapMotorOff", "SR-ID-IU22B-25:gapMotorOff", "SR-ID-EPU48A-41:gapMotorOff", "SR-ID-EPU48B-41:gapMotorOff", "SR-ID-EPU46-45:gapMotorOff", "SR-ID-EPU48A-41:phaseMotorOff", "SR-ID-EPU48B-41:phaseMotorOff", "SR-ID-EPU46-45:phaseMotorOff"]) -> ("1rst Value (string)"=w50:string[])  [unwired: 8 in, 6 out]
  n45 = Get Date/Time In Seconds() -> (seconds since 1Jan1904=w15:timestamp)
  n46 = for {
    tunnel: w50 -> [w338] mode=indexing
    tunnel: [w337] -> w49 mode=indexing
    n47 = case shown="\"0\"" w338 {
      tunnel: [FALSE TRUE] -> w337
      frame "1", Default {
      }
      frame "0" {
      }
    }
  }
  n48 = call-poly <userlib>:"CaLabGet.vi"("PV Names"=string[] ["FE-DI-XBPM-051:SA:SA_X_MONITOR", "FE-DI-XBPM-051:SA:SA_Y_MONITOR", "FE-DI-XBPM-091:SA:SA_X_MONITOR", "FE-DI-XBPM-091:SA:SA_Y_MONITOR", "FE-DI-XBPM-211:SA:SA_X_MONITOR", "FE-DI-XBPM-211:SA:SA_Y_MONITOR", "FE-DI-XBPM-231:SA:SA_X_MONITOR", "FE-DI-XBPM-231:SA:SA_Y_MONITOR", "FE-DI-XBPM-251:SA:SA_X_MONITOR", "FE-DI-XBPM-251:SA:SA_Y_MONITOR", "FE-DI-XBPM-411:SA:SA_X_MONITOR", "FE-DI-XBPM-411:SA:SA_Y_MONITOR", "FE-DI-XBPM-451:SA:SA_X_MONITOR", "FE-DI-XBPM-451:SA:SA_Y_MONITOR"]) -> ("1rst Value (number)"=w66:dbl[])  [unwired: 8 in, 6 out]
  n49 = call-poly <userlib>:"CaLabGet.vi"("PV Names"=w5) -> ("1rst Value (number)"=w7:dbl[])  [unwired: 8 in, 6 out]
  n50 = call-poly <userlib>:"CaLabGet.vi"("PV Names"=w6) -> ("1rst Value (number)"=w10:dbl[])  [unwired: 8 in, 6 out]
  n51 = Format Date/Time String(time format string (%c)="%Y\\%m\\%d", seconds (now)=w15) -> ()  [unwired: 1 in, 1 out]
  n52 = Format Date/Time String(time format string (%c)="%Y/%m/%d", seconds (now)=w15) -> (date/time string=→"date":string)  [unwired: 1 in]
  n53 = Format Date/Time String(time format string (%c)="%H:%M:%S", seconds (now)=w15) -> (date/time string=→"time string":string)  [unwired: 1 in]
  n54 = Multiply(x=w66, y=0.01) -> (x*y=w65:dbl[])
  "Value Array (number) 7" <- w65
  n55 = Multiply(x=w7, y=w9) -> (x*y=w8:dbl[])
  n56 = Index Array(array=w65, index #1=0 ("index"), index #2=1 ("index"), index #3=2 ("index"), index #4=3 ("index"), index #5=4 ("index"), index #6=5 ("index"), index #7=6 ("index"), index #8=7 ("index"), index #9=8 ("index"), index #10=9 ("index"), index #11=10 ("index"), index #12=11 ("index"), index #13=12 ("index"), index #14=13 ("index")) -> (element #1=→"05XBPMX 1":dbl, element #2=→"05XBPMY 1":dbl, element #3=→"09XBPMX 1":dbl, element #4=→"09XBPMY 1":dbl, element #5=→"21XBPMX 1":dbl, element #6=→"21XBPMY 1":dbl, element #7=→"23XBPMX 1":dbl, element #8=→"23XBPMY 1":dbl, element #9=→"25XBPMX 1":dbl, element #10=→"25XBPMY 1":dbl, element #11=→"41XBPMX 1":dbl, element #12=→"41XBPMY 1":dbl, element #13=→"45XBPMX 1":dbl, element #14=→"45XBPMY 1":dbl)
  n57 = Multiply(x=w10, y=w9) -> (x*y=w11:dbl[])
  n58 = call-poly <userlib>:"CaLabGet.vi"("PV Names"=w136) -> ("1rst Value (string)"=w144:string[])  [unwired: 8 in, 6 out]
  n59 = for {
    tunnel: w144 -> [w342] mode=indexing
    tunnel: [w341] -> w145 mode=indexing
    n60 = case shown="\"Enable\"" w342 {
      tunnel: [FALSE TRUE] -> w341
      frame "Disable", Default {
      }
      frame "Enable" {
      }
    }
  }
  n61 = Index Array(array=w49, index #1=0 ("index"), index #2=1 ("index"), index #3=2 ("index"), index #4=3 ("index"), index #5=4 ("index"), index #6=5 ("index"), index #7=6 ("index"), index #8=7 ("index"), index #9=8 ("index"), index #10=9 ("index"), index #11=10 ("index"), index #12=11 ("index"), index #13=12 ("index")) -> (element #1=→"IU22-05M":bool, element #2=→"IU22A-09M":bool, element #3=→"IU22B-09M":bool, element #4=→"IUT22-21M":bool, element #5=→"IU22-23M":bool, element #6=→"IU22A-25M":bool, element #7=→"IU22B-25M":bool, element #8=→"EPU48A-41gM":bool, element #9=→"EPU48A-41pM":bool, element #10=→"EPU48B-41gM":bool, element #11=→"EPU48B-41pM":bool, element #12=→"EPU46-45gM":bool, element #13=→"EPU46-45pM":bool)
  n62 = call-poly <userlib>:"CaLabGet.vi"("PV Names"=w162) -> ("1rst Value (string)"=w154:string[])  [unwired: 8 in, 6 out]
  n63 = for {
    tunnel: w154 -> [w346] mode=indexing
    tunnel: [w345] -> w153 mode=indexing
    n64 = case shown="\"disable\", Default" w346 {
      tunnel: [FALSE TRUE] -> w345
      frame "disable", Default {
      }
      frame "enable" {
      }
    }
  }
  n65 = call-poly <userlib>:"CaLabGet.vi"("PV Names"=string[] ["SR-ID-IU22-05:getGap", "SR-ID-IU22A-09:getGap", "SR-ID-IU22B-09:getGap", "SR-ID-IUT22-21:getGap", "SR-ID-IU22-23:getGap", "SR-ID-IU22A-25:getGap", "SR-ID-IU22B-25:getGap", "SR-ID-EPU48A-41:getGap", "SR-ID-EPU48A-41:getPhase", "SR-ID-EPU48B-41:getGap", "SR-ID-EPU48B-41:getPhase", "SR-ID-EPU46-45:getGap", "SR-ID-EPU46-45:getPhase", "SR-ID-IUT22-21:getGapTaper", "SR-ID-EPU48PS-41:getGap"]) -> ("1rst Value (number)"=w128:dbl[])  [unwired: 8 in, 6 out]
  "Value Array (number) 6" <- w128
  n66 = Bundle("Array 4"=w12, w8) -> (→"BPMX Graph":cluster{"Array 4":i32[], dbl[]})  [unwired: 1 in]
  n67 = Bundle("Array 4"=w12, w11) -> (→"BPMY Graph":cluster{"Array 4":i32[], dbl[]})  [unwired: 1 in]
  n68 = Index Array(array=w128, index #1=0 ("index"), index #2=1 ("index"), index #3=2 ("index"), index #4=3 ("index"), index #5=4 ("index"), index #6=5 ("index"), index #7=6 ("index"), index #8=7 ("index"), index #9=8 ("index"), index #10=9 ("index"), index #11=10 ("index"), index #12=11 ("index"), index #13=12 ("index"), index #14=13 ("index"), index #15=14 ("index")) -> (element #1=→"IU22-05gap(R)":dbl, element #2=→"IU22A-09gap(R)":dbl, element #3=→"IU22B-09gap(R)":dbl, element #4=→"IUT22-21gap(R)":dbl, element #5=→"IU22-23gap(R)":dbl, element #6=→"IU22A-25gap(R)":dbl, element #7=→"IU22B-25gap(R)":dbl, element #8=→"EPU48A-41gap(R)":dbl, element #9=→"EPU48A-41phase(R)":dbl, element #10=→"EPU48B-41gap(R)":dbl, element #11=→"EPU48B-41phase(R)":dbl, element #12=→"EPU46-45gap(R)":dbl, element #13=→"EPU46-45phase(R)":dbl, element #14=→"Taper":dbl, element #15=→"phase shifter":dbl)
  n69 = Index Array(array=w145, index #1=0 ("index"), index #2=1 ("index"), index #3=2 ("index"), index #4=3 ("index"), index #5=4 ("index"), index #6=5 ("index"), index #7=6 ("index")) -> (element #1=→"IU22-05 Hutch Enable":bool, element #2=→"IU22A-09M Hutch Enable":bool, element #3=→"IUT22-21M Hutch Enable":bool, element #4=→"IU22-23M Hutch Enable":bool, element #5=→"IU22A-25M Hutch Enable":bool, element #6=→"EPU48A-41M Hutch Enable":bool, element #7=→"EPU46-45M Hutch Enable":bool)
  n70 = Index Array(array=w153, index #1=0 ("index"), index #2=1 ("index"), index #3=2 ("index"), index #4=3 ("index"), index #5=4 ("index"), index #6=5 ("index"), index #7=6 ("index")) -> (element #1=→"IU22-05 FE Enable":bool, element #2=→"IU22A-09 FE Enable":bool, element #3=→"IUT22-21 FE Enable":bool, element #4=→"IU22-23 FE Enable":bool, element #5=→"IU22A-25 FE Enable":bool, element #6=→"EPU48A-41 FE Enable":bool, element #7=→"EPU46-45 FE Enable":bool)
  n71 = call-poly <userlib>:"CaLabGet.vi"("PV Names"=string[] ["SR-DI-FOFB-H:getStatus", "SR-DI-FOFB-V:getStatus", "IGPF:TPSX:FBCTRL", "IGPF:TPSY:FBCTRL", "TPS-SR-052:bpm4:ilk:enabled", "SR-DI-ANGLE-ILK:StatusX", "SR-DI-ANGLE-ILK:StatusY"]) -> ("1rst Value (string)"=w31:string[], "1rst Value (number)"=w28:dbl[])  [unwired: 8 in, 5 out]
  n72 = To Byte Integer(number=w28) -> (8bit integer=w34:i8[])
  n73 = for {
    tunnel: w34 -> [w350] mode=indexing
    tunnel: [w349] -> w22 mode=indexing
    n74 = case shown="1" w350 {
      tunnel: [TRUE FALSE] -> w349
      frame 1 {
      }
      frame 0, Default {
      }
    }
  }
  n75 = Index Array(array=w31, index #1=0 ("index"), index #2=1 ("index")) -> (element #1=→"FOFB H":string, element #2=→"FOFB V":string)
  n76 = Index Array(array=w22, index #1=2 ("index"), index #2=3 ("index"), index #3=4 ("index"), index #4=5 ("index"), index #5=6 ("index")) -> (element #1=→"BBF H":bool, element #2=→"BBF V":bool, element #3=→"Orbit ILK(P)":bool)  [unwired: 2 out]
